vi "Element Type.vi"(11 "BooleanControl in":refnum<class "BooleanControl.lvclass">) -> (2 "Element Type":string)   [LabVIEW 2020, in "VolatusGUIElements.lvlib" / "BooleanControl.lvclass"]
uses:
  BooleanControl.lvclass
  BooleanControl.lvclass/BooleanControl.ctl
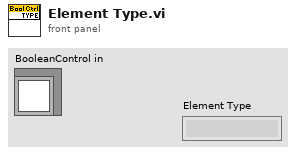
[diagram p1: front panel]
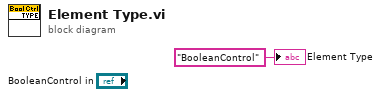
[diagram p0: block diagram]
diagram:
  "Element Type" <- "BooleanControl" ("Element Type")
